vi "Execute 7z bat.vi"(8 "error in (no error)":errorcluster, 11 "source path":path=path "C:/user/patrick/git/Multichannel-Lockin/src") -> (0 "error out":errorcluster)   [LabVIEW 2016]
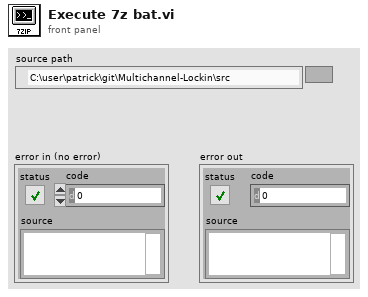
[diagram p1: front panel]
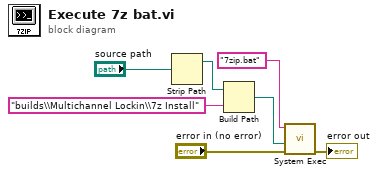
[diagram p0: block diagram]
diagram:
  n1 = Strip Path(path="source path") -> (stripped path=w4:path)  [unwired: 1 out]
  n2 = Build Path(base path=w4, name or relative path="builds\\Multichannel Lockin\\7z Install") -> (appended path=w2:path)
  n3 = call <vilib>:"System Exec.vi"("error in (no error)"="error in (no error)", "working directory"=w2, "command line"="7zip.bat" ("name or relative path")) -> ("error out"=→"error out":errorcluster)  [unwired: 5 in, 3 out]
